vi "sub_omega tasks.vi"(5 "DAQ Channel":string, 6 "Omega errors":errorcluster[](array[cluster]), 9 "Omega tasks":refnum<k24>[](array[refnum])) -> (0 "Omega errors out":errorcluster[](array[cluster]), 3 "Omega tasks out":refnum<k24>[](array[refnum]), 4 "Source Number":i32)   [LabVIEW 2021]
uses:
  <vilib>/ULx/ULx_LV.dll
  <vilib>/ULx/Create Channel.llb/ULx Create Channel (AI-Temperature).vi
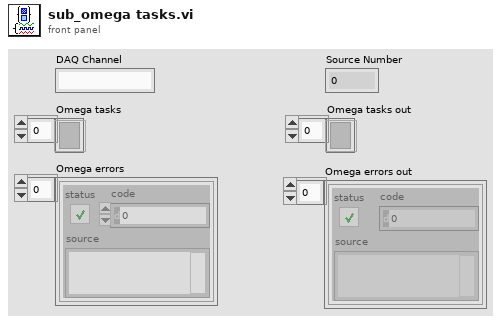
[diagram p1: front panel]
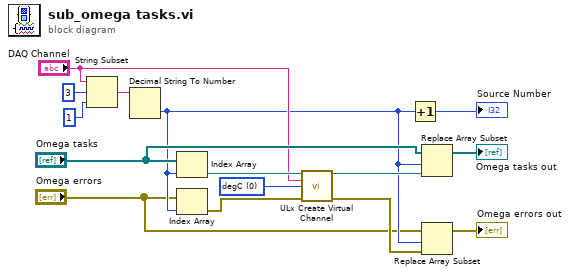
[diagram p0: block diagram]
diagram:
  w1 = 0 items=["degC", "degF", "kelvin", "raw"] ("units")
  n1 = String Subset(string="DAQ Channel", offset (0)=3, length (rest)=1) -> (substring=w11:string)
  n2 = Decimal String To Number(string=w11) -> (number=w4:i32)  [unwired: 2 in, 1 out]
  n3 = Index Array(array="Omega tasks", index=w4) -> (element=w12:refnum<k24>)
  n4 = Index Array(array="Omega errors", index=w4) -> (element=w6:errorcluster)
  n5 = call-poly <vilib>:"ULx Create Virtual Channel.vi"("task in"=w12, "physical channels"="DAQ Channel", "units"=w1, "error in"=w6) -> ("task out"=w13:refnum<k24>, "error out"=w5:errorcluster)  [unwired: 10 in]
  n6 = Increment(x=w4) -> (x+1=→"Source Number":i32)
  n7 = Replace Array Subset(array="Omega tasks", new element=w13, index=w4) -> (→"Omega tasks out":refnum<k24>[])
  n8 = Replace Array Subset(array="Omega errors", new element=w5, index=w4) -> (→"Omega errors out":errorcluster[])
